vi "Init Rx - Execution Details.vi"(8 "error in (no error)":errorcluster, 11 "Rx Loop Data in":T1) -> (0 "error out":errorcluster, 2 "Target Processor":i32, 3 "Rx Loop Data out":T1, 5 "Priority":i32)   [LabVIEW 2016, in "UDP-Custom-Device Engine.lvlib"]
uses:
  UDP-Custom-Device Engine.lvlib
  Types/Engine - Rx Loop Data.ctl
  <vilib>/NI Veristand/VeriStand Data/Byte Buffer/Byte Buffer.lvclass
  Types/Engine - General Resources.ctl
  <vilib>/NI Veristand/VeriStand Data/Typedefs/Typedefs.Data Types.ctl
  Shared/Types/Shared - Duplex Settings.ctl
  Shared/Types/Shared - Header Details.ctl
  Types/Engine - Data Conversion Config.ctl
  <vilib>/NI Veristand/VeriStand Data/Byte Buffer/Byte Buffer.Mapping.ctl
  Types/Engine - Rx Runtime Resources.ctl
  Types/Engine - Rx New Data Options Support.ctl
  Shared/Types/Shared - New Data Options.ctl
  Types/Engine - Rx Channel Refs.ctl
  <vilib>/NI/NIVS Inline Async API/_Data Access Engine/Data Access Engine/Types/Write.DVR.ctl
  <vilib>/NI/NIVS Inline Async API/_Data Access Engine/Access Type Classes/Write/Write.lvclass
  Types/Engine - Debug Resources.ctl
  <vilib>/NI Veristand/VeriStand Data/VeriStand Data.lvlib
  Shared/UDP-Custom-Device Shared.lvlib
  <vilib>/NI/NIVS Inline Async API/_Data Access Engine/Data Access Engine/Data Access Engine.lvclass
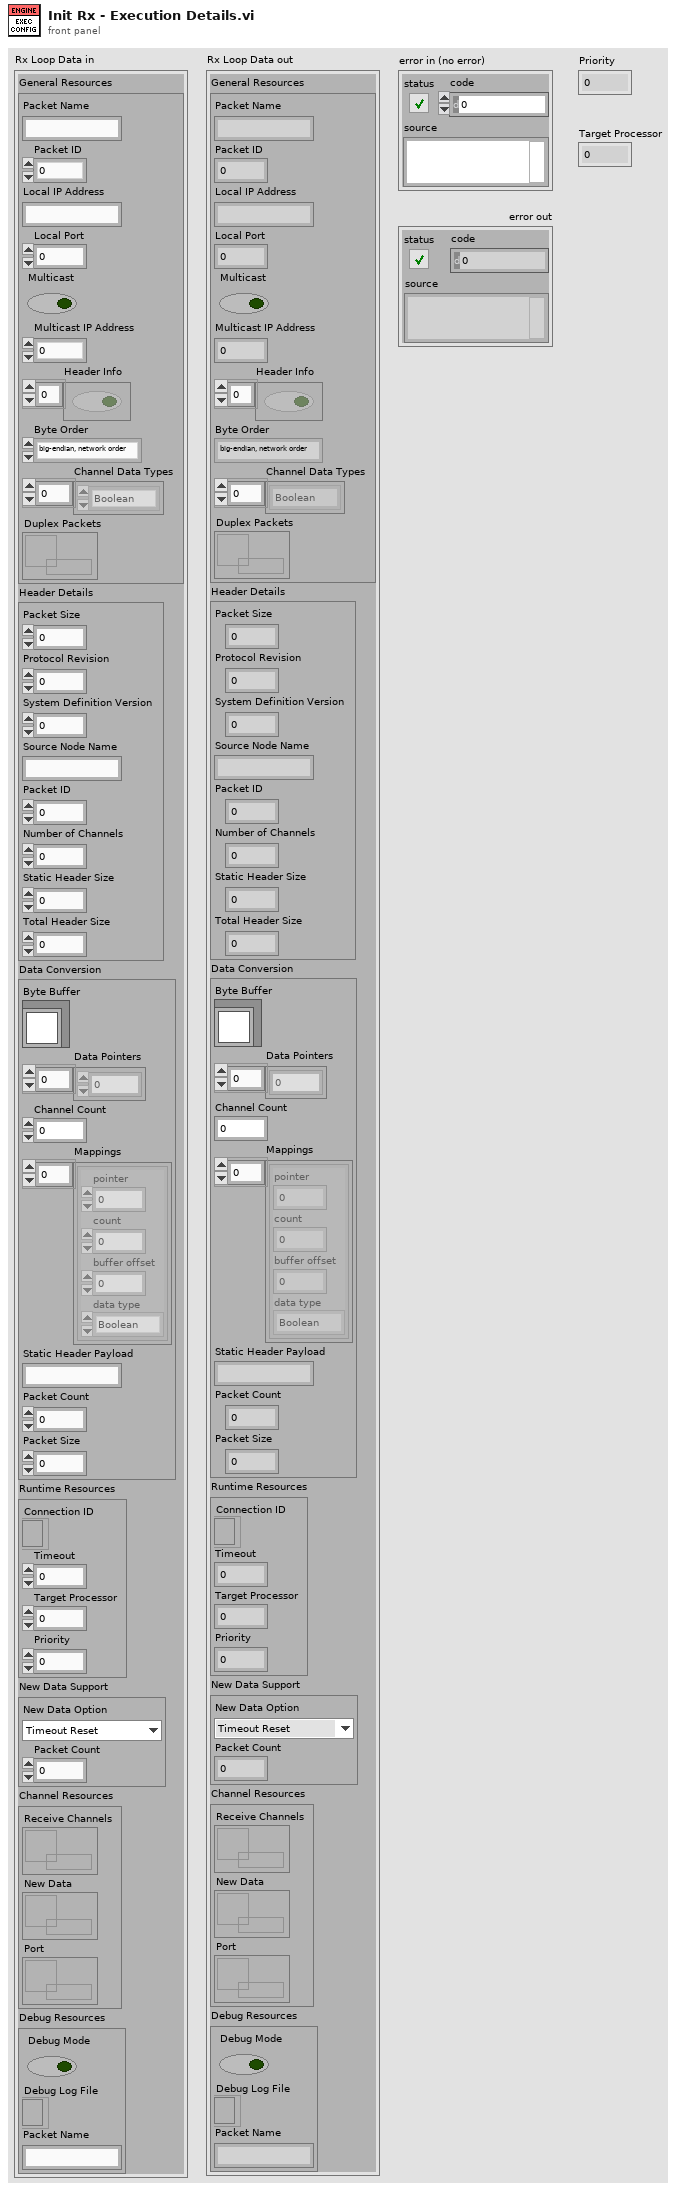
[diagram p1: front panel]
types:
  T1 = typedef "UDP-Custom-Device Engine.lvlib/Engine - Rx Loop Data.ctl" = cluster{"General Resources":T2, "Header Details":T4, "Data Conversion":T5, "Runtime Resources":T7, "New Data Support":T8, "Channel Resources":T10, "Debug Resources":T12}
  T2 = typedef "UDP-Custom-Device Engine.lvlib/Engine - General Resources.ctl" = cluster{"Packet Name":string, "Packet ID":i32, "Local IP Address":string, "Local Port":i32, "Multicast":bool, "Multicast IP Address":u32, "Header Info":bool[], "Byte Order":enum16{"big-endian, network order", "native, host order", "little-endian"}, "Channel Data Types":T3[], "Duplex Packets":refnum<data-value>}
  T3 = typedef "VeriStand Data.lvlib/Typedefs.Data Types.ctl" = enum16{"Boolean", "Single", "Double", "I8", "I16", "I32", "I64", "U8", "U16", "U32", "U64"}
  T4 = typedef "UDP-Custom-Device Shared.lvlib/Shared - Header Details.ctl" = cluster{"Packet Size":u16, "Protocol Revision":u8, "System Definition Version":u64, "Source Node Name":string, "Packet ID":u32, "Number of Channels":u32, "Static Header Size":u16, "Total Header Size":u16}
  T5 = typedef "UDP-Custom-Device Engine.lvlib/Engine - Data Conversion Config.ctl" = cluster{"Byte Buffer":refnum<class "Byte Buffer.lvclass">, "Data Pointers":u64[], "Channel Count":i32, "Mappings":T6[], "Static Header Payload":string, "Packet Count":dbl, "Packet Size":i32}
  T6 = typedef "VeriStand Data.lvlib/Byte Buffer.lvclass/Byte Buffer.Mapping.ctl" = cluster{"pointer":u64, "count":i64, "buffer offset":u64, "data type":T3}
  T7 = typedef "UDP-Custom-Device Engine.lvlib/Engine - Rx Runtime Resources.ctl" = cluster{"Connection ID":refnum<k16>, "Timeout":i32, "Target Processor":i32, "Priority":i32}
  T8 = typedef "UDP-Custom-Device Engine.lvlib/Engine - Rx New Data Options Support.ctl" = cluster{"New Data Option":T9, "Packet Count":dbl}
  T9 = typedef "UDP-Custom-Device Shared.lvlib/Shared - New Data Options.ctl" = enum16{"Timeout Reset", "Counter"}
  T10 = typedef "UDP-Custom-Device Engine.lvlib/Engine - Rx Channel Refs.ctl" = cluster{"Receive Channels":T11, "New Data":T11, "Port":T11}
  T11 = typedef "Data Access Engine.lvlib/Data Access Engine.lvclass/Write.DVR.ctl" = refnum<data-value>
  T12 = typedef "UDP-Custom-Device Engine.lvlib/Engine - Debug Resources.ctl" = cluster{"Debug Mode":bool, "Debug Log File":refnum<file>, "Packet Name":string}
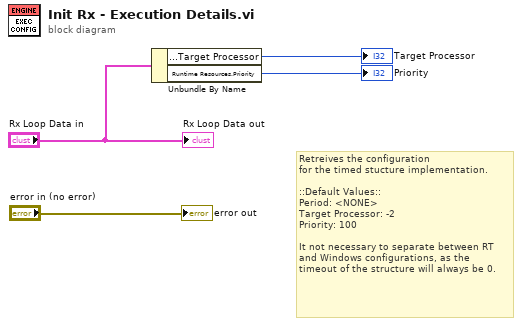
[diagram p0: block diagram]
diagram:
  # "Retreives the configuration\nfor the timed stucture implementation.\n\n::Default Values::\nPeriod: <NONE>\nTarget Processor: -2\nPriority: 100\n\nIt not necessary to separate between RT\nand Windows configurations, as the\ntimeout of the structure will always be 0."
  n1 = Unbundle By Name("Rx Loop Data in") -> ("Runtime Resources.Target Processor"=→"Target Processor":i32, "Runtime Resources.Priority"=→"Priority":i32)
  "Rx Loop Data out" <- "Rx Loop Data in"
  "error out" <- "error in (no error)"
